vi "XNET UDP Socket Write.vi"   [LabVIEW 2018]
doc: "Writes a datagram to a remote UDP port. To send multicast datagrams, specify the multicast group address in the remote address input."
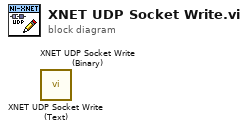
[diagram p0: block diagram]
diagram:
  n1 = call "XNET UDP Socket Write (Text).vi"() -> ()  [unwired: 10 in, 2 out]
  n2 = call "XNET UDP Socket Write (Binary).vi"() -> ()  [unwired: 10 in, 2 out]
